vi "Create Framework.vi"(8 "error in (no error)":errorcluster, 11 "Application Data in":T1) -> (0 "error out":errorcluster, 2 "new item tag":string, 3 "Application Data Out":T1)   [LabVIEW 2017, in "DSF Data Viewer.lvlib"]
uses:
  DSF Data Viewer.lvlib
  Main VI/Application Data.ctl
  <vilib>/NI/Memory Manager/Classes/Pointer/Pointer.lvclass
  Builds/Data Sharing Framework/Current/Core/DSF Core.lvlibp/Engine/Classes/Framework/Framework.lvclass
  Buffer Reader/Buffer Data.ctl
  Builds/Data Sharing Framework/Current/Core/DSF Core.lvlibp/Engine/Classes/Buffer/Buffer.lvclass
  Builds/Data Sharing Framework/Current/Core/DSF Core.lvlibp/Engine/Classes/Transfer Group Status/Transfer Group Status.lvclass
  ID to Tree Items/Tree Item Type.ctl
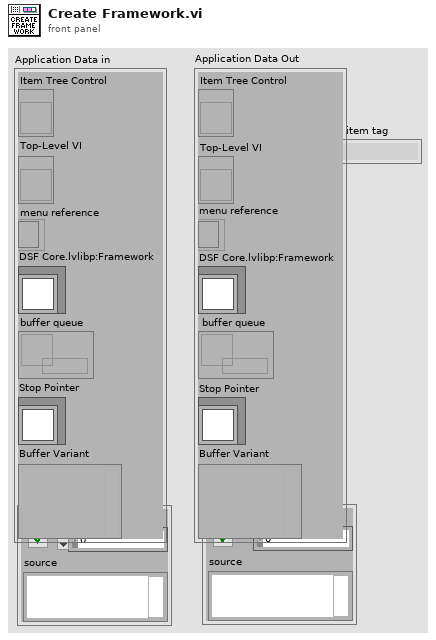
[diagram p1: front panel]
types:
  T1 = typedef "DSF Data Viewer.lvlib/Application Data.ctl" = cluster{"Item Tree Control":refnum<vi>, "Top-Level VI":refnum<vi>, "menu reference":refnum<k9>, "DSF Core.lvlibp:Framework":refnum<class "Framework.lvclass">, "buffer queue":refnum<queue>, "Stop Pointer":refnum<class "Pointer.lvclass">, "Buffer Variant":variant}
  T2 = typedef "DSF Data Viewer.lvlib/Buffer Data.ctl" = cluster{"DSF Core.lvlibp:Buffer":refnum<class "Buffer.lvclass">, "DSF Core.lvlibp:Transfer Group Status.lvclass":refnum<class "Transfer Group Status.lvclass">, "decimation":u64}
  T3 = typedef "DSF Data Viewer.lvlib/Tree Item Type.ctl" = enum16{"Framework", "Plugin Group", "Plugin", "Group", "Transfer", "Buffer", "Channel"}
  T4 = typedef "DSF Data Viewer.lvlib/Tree Item.ctl" = cluster{"Left Cell String":string, "Child Text":string[], "Child Tag":string, "Glyph Index":i32}
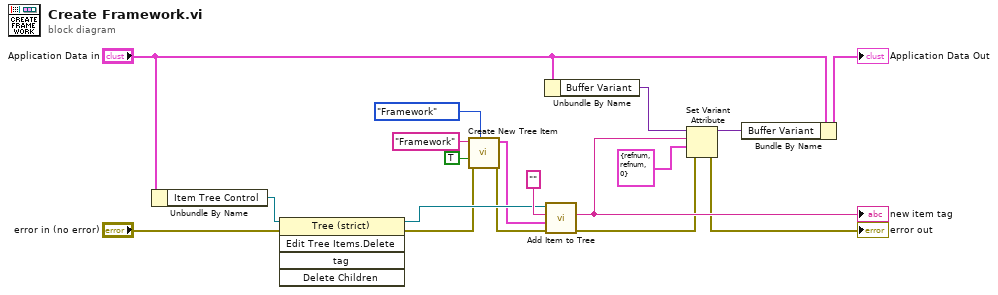
[diagram p0: block diagram]
diagram:
  n1 = Unbundle By Name("Application Data in") -> ("Item Tree Control"=w10:refnum<vi>)
  n2 = invoke class="Tree (strict)" method="Edit Tree Items.Delete"(reference=w10, error in="error in (no error)") -> (reference out=w17:refnum<vi>, error out=w16:errorcluster)  [unwired: 3 in, 3 out]
  n3 = call "Create New Tree Item.vi"("Item Type"=Tree_Item_Type."Framework", "error in"=w16, "found?"=TRUE, "Left Cell String"="Framework") -> ("error out"=w15:errorcluster, "Item"=w14:T4)  [unwired: 6 in]
  n4 = Unbundle By Name("Application Data in") -> ("Buffer Variant"=w7:variant)
  n5 = call "Add Item to Tree.vi"("error in (no error)"=w15, "Item"=w14, "parent tag"="", "TreeControl in"=w17) -> ("error out"=w6:errorcluster, "new item tag"=w8:string)  [unwired: 5 in, 1 out]
  "new item tag" <- w8
  n6 = Set Variant Attribute(Variant=w7, name=w8, value=T2 {"DSF Core.lvlibp:Buffer"=refnum, "DSF Core.lvlibp:Transfer Group Status.lvclass"=refnum, "decimation"=0} ("Buffer data"), error in=w6) -> (Variant out=w3:variant, error out=→"error out":errorcluster)  [unwired: 1 out]
  n7 = Bundle By Name(cluster="Application Data in", "Buffer Variant"=w3) -> (→"Application Data Out":T1)
